vi "Validate Video Prefs.vi"(8 "error in (no error)":errorcluster, 10 "Video Prefs":T1, 11 "SB App in":refnum<class "SB App.lvclass">) -> (0 "error out":errorcluster, 2 "Valid?":bool, 3 "SB App out":refnum<class "SB App.lvclass">)   [LabVIEW 2020, in "SB App.lvlib" / "SB App.lvclass"]
uses:
  SB App.lvclass
  SB App.lvclass/SB App.ctl
  Video Prefs.ctl
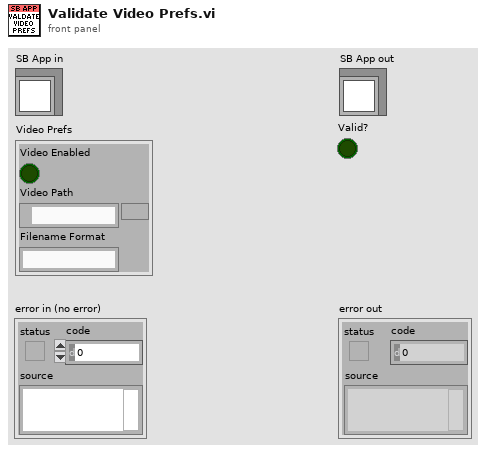
[diagram p1: front panel]
types:
  T1 = typedef "SB App.lvlib/SB App.lvclass/Video Prefs.ctl" = cluster{"Video Enabled":bool, "Video Path":path, "Filename Format":string}
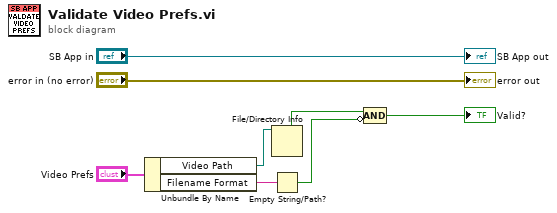
[diagram p0: block diagram]
diagram:
  n1 = Unbundle By Name("Video Prefs") -> ("Video Path"=w5:path, "Filename Format"=w4:string)
  n2 = File/Directory Info(path=w5) -> (directory=w3:bool)  [unwired: 1 in, 6 out]
  n3 = Empty String/Path?(string/path=w4) -> (empty?=w2:bool)
  n4 = Compound Arithmetic op=AND(w3, invert w2) -> (→"Valid?":bool)
  "error out" <- "error in (no error)"
  "SB App out" <- "SB App in"
